vi "VariantToByteArray.vi"(8 "error in":errorcluster, 9 "bytearray_in":u8[](array[numeric]), 11 "variant":variant) -> (0 "error out":errorcluster, 3 "byte_array_out[]":u8[](array[numeric]))   [LabVIEW 2020]
uses:
  <vilib>/Utility/Data Type/NI_Data Type.lvlib
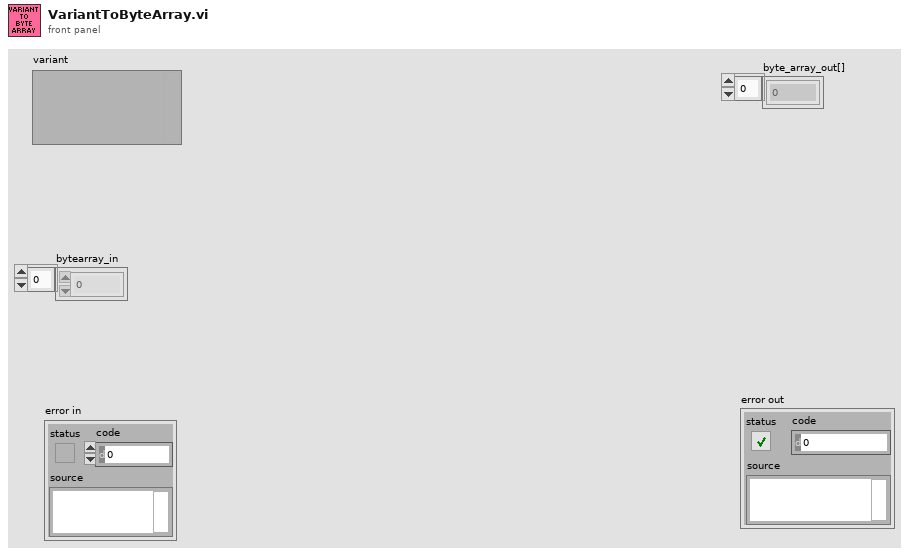
[diagram p1: front panel]
types:
  T1 = typedef "NI_Data Type.lvlib/Data Type.ctl" = enum8{"Invalid Type", "Void", "I8", "I16", "I32", "I64", "U8", "U16", "U32", "U64", "Single Float", "Double Float", "Extended Float", "Single Complex", "Double Complex", "Extended Complex", "Enum U8", "Enum U16", "Enum U32", "Enum U64", "Single Float With Unit", "Double Float With Unit", "Extended Float With Unit", "Single Complex with Unit", "Double Complex with Unit", "Extended Complex with Unit", "Boolean", "String", "Path", "Picture", "Tag", "Array", "Cluster", "Variant", "LV Variant", "Waveform", "Timestamp", "Digital Waveform", "Digital Data", "ExpressData", "Refnum", "External Data", "VI", "Poly VI", "LabVIEW Class Instance", "Fixed Point", "Set Collection", "Map Collection"}
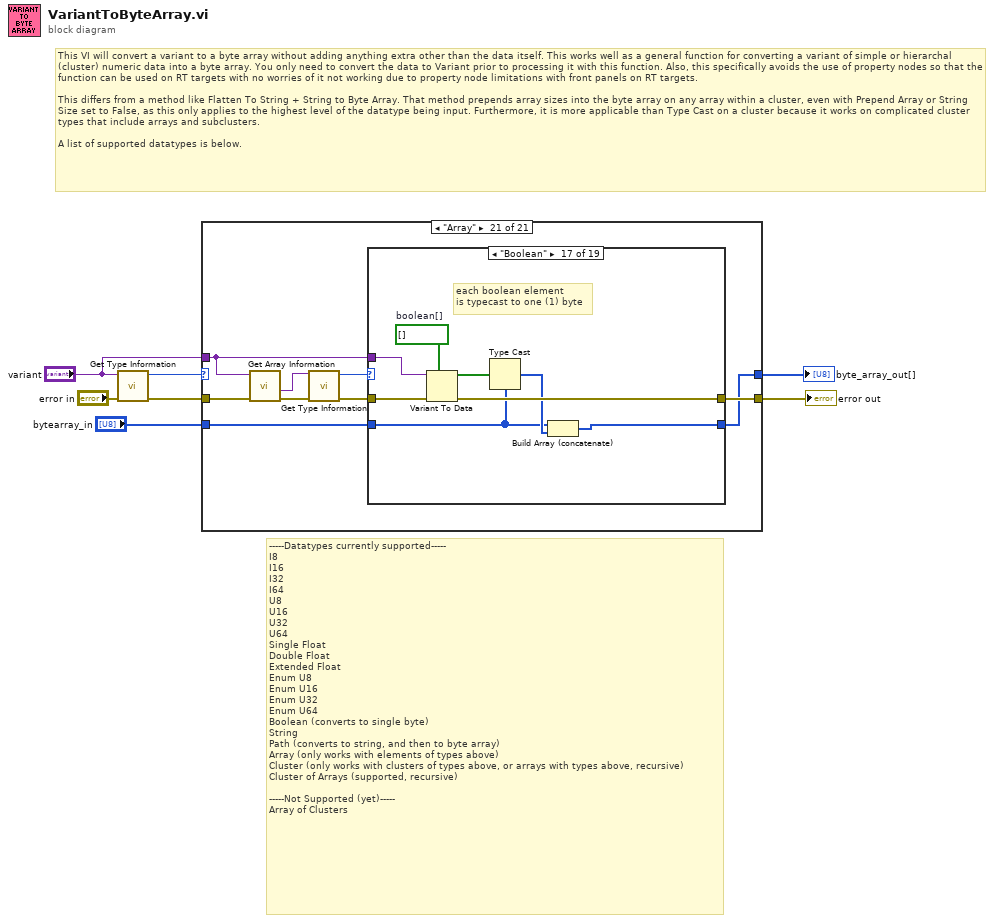
[diagram p0: block diagram]
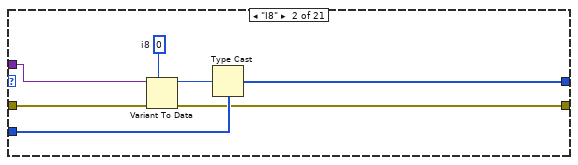
[diagram p3: hidden frame]
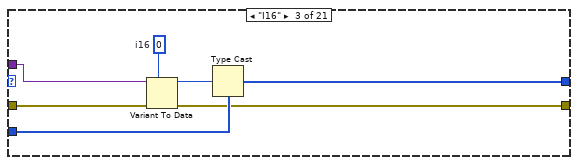
[diagram p4: hidden frame]
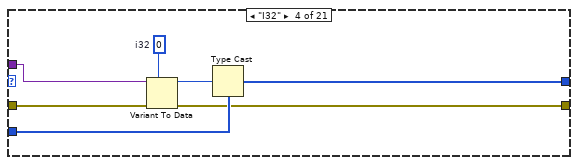
[diagram p5: hidden frame]
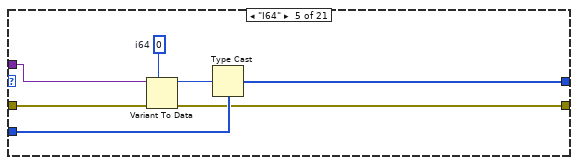
[diagram p6: hidden frame]
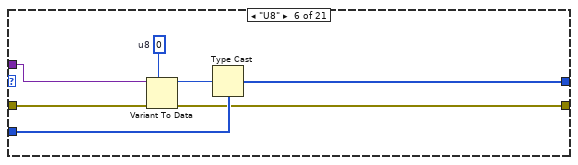
[diagram p7: hidden frame]
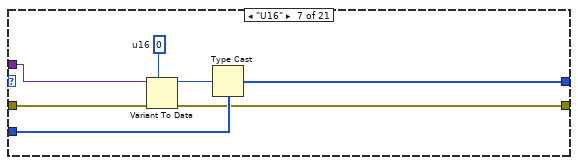
[diagram p8: hidden frame]
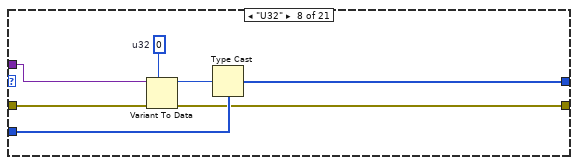
[diagram p9: hidden frame]
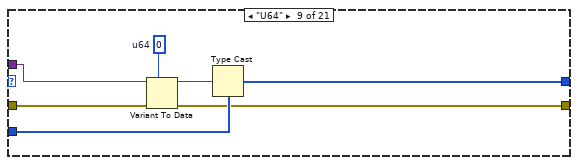
[diagram p10: hidden frame]
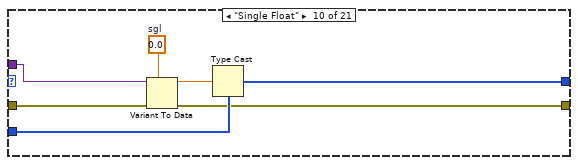
[diagram p11: hidden frame]
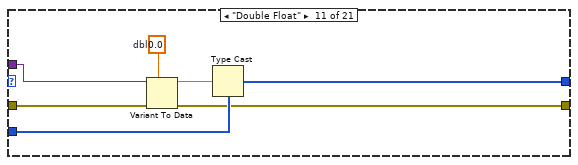
[diagram p12: hidden frame]
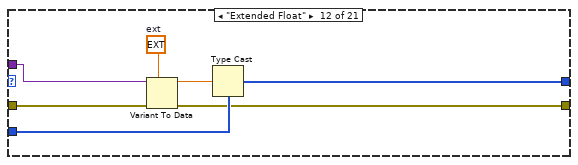
[diagram p13: hidden frame]
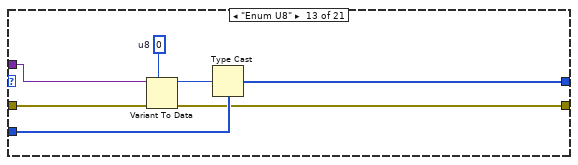
[diagram p14: hidden frame]
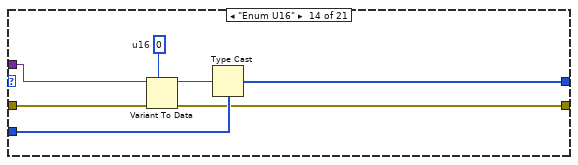
[diagram p15: hidden frame]
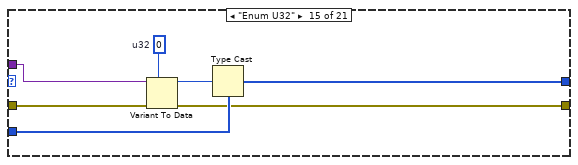
[diagram p16: hidden frame]
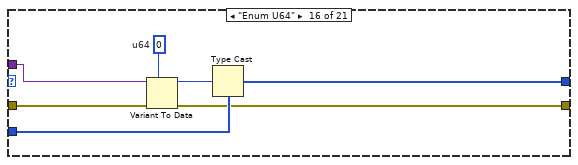
[diagram p17: hidden frame]
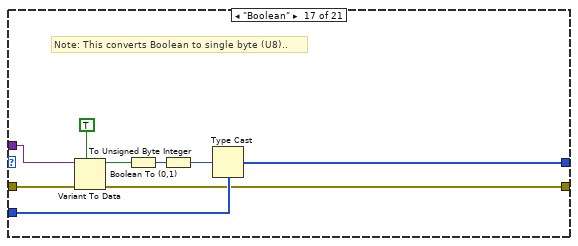
[diagram p18: hidden frame]
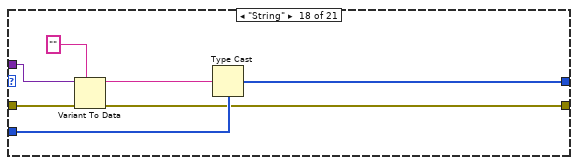
[diagram p19: hidden frame]
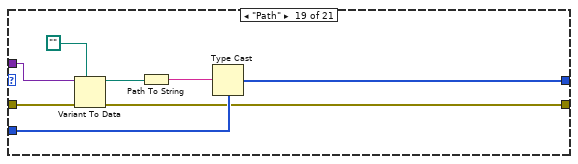
[diagram p20: hidden frame]
diagram:
  # "This VI will convert a variant to a byte array without adding anything extra other than the data itself. This works well as a general function for converting a variant of simple or hierarchal (cluster) numeric data into a byte array. You only need to convert the data to Variant prior to processing it with this function. Also, this specifically avoids the use of property nodes so that the function can be used on RT targets with no worries of it not working due to property node limitations with front panels on RT targets.\n\nThis differs from a method like Flatten To String + String to Byte Array. That method prepends array sizes into the byte array on any array within a cluster, even with Prepend Array or String Size set to False, as this only applies to the highest level of the datatype being input. Furthermore, it is more applicable than Type Cast on a cluster because it works on complicated cluster types that include arrays and subclusters.\n\nA list of supported datatypes is below."
  # "-----Datatypes currently supported-----\nI8\nI16\nI32\nI64\nU8\nU16\nU32\nU64\nSingle Float\nDouble Float\nExtended Float\nEnum U8\nEnum U16\nEnum U32\nEnum U64\nBoolean (converts to single byte)\nString\nPath (converts to string, and then to byte array)\nArray (only works with elements of types above)\nCluster (only works with clusters of types above, or arrays with types above, recursive) \nCluster of Arrays (supported, recursive)\n\n-----Not Supported (yet)-----\nArray of Clusters"
  n1 = call <vilib>:"Get Type Information.vi"("error in (no error)"="error in", "variant"="variant") -> ("error out"=w6:errorcluster, "type"=w7:T1)  [unwired: 5 in, 3 out]
  n2 = case shown="\"Array\"" w7 {
    tunnel: "variant" -> [_ w16 w23 w30 w37 w44 w51 w58 w65 w72 w79 w86 w93 w100 w107 w114 w123 w130 w138 w145 w155]
    tunnel: [w8 w13 w20 w27 w34 w41 w48 w55 w62 w69 w76 w83 w90 w97 w104 w111 w121 w129 w137 w140 w154] -> w1
    tunnel: "bytearray_in" -> [w8 w12 w19 w26 w33 w40 w47 w54 w61 w68 w75 w82 w89 w96 w103 w110 w120 w128 w136 w141 w157]
    tunnel: w6 -> [w9 w11 w18 w25 w32 w39 w46 w53 w60 w67 w74 w81 w88 w95 w102 w109 w119 w127 w135 w144 w161]
    tunnel: [w9 w10 w17 w24 w31 w38 w45 w52 w59 w66 w73 w80 w87 w94 w101 w108 w118 w126 w134 w139 w162] -> w2
    frame "Invalid Type", Default {
    }
    frame "I8" {
      w14 = i8 0  # i8
      n3 = Variant To Data(error in=w11, type=w14, Variant=w16) -> (data=w15:i8, error out=w10:errorcluster)
      n4 = Type Cast(type=w12, x=w15) -> (*(type *) &x=w13:u8[])
    }
    frame "I16" {
      w21 = i16 0  # i16
      n5 = Variant To Data(error in=w18, type=w21, Variant=w23) -> (data=w22:i16, error out=w17:errorcluster)
      n6 = Type Cast(type=w19, x=w22) -> (*(type *) &x=w20:u8[])
    }
    frame "I32" {
      w28 = 0  # i32
      n7 = Variant To Data(error in=w25, type=w28, Variant=w30) -> (data=w29:i32, error out=w24:errorcluster)
      n8 = Type Cast(type=w26, x=w29) -> (*(type *) &x=w27:u8[])
    }
    frame "I64" {
      w35 = i64 0  # i64
      n9 = Variant To Data(error in=w32, type=w35, Variant=w37) -> (data=w36:i64, error out=w31:errorcluster)
      n10 = Type Cast(type=w33, x=w36) -> (*(type *) &x=w34:u8[])
    }
    frame "U8" {
      w42 = u8 0  # u8
      n11 = Variant To Data(error in=w39, type=w42, Variant=w44) -> (data=w43:u8, error out=w38:errorcluster)
      n12 = Type Cast(type=w40, x=w43) -> (*(type *) &x=w41:u8[])
    }
    frame "U16" {
      w49 = u16 0  # u16
      n13 = Variant To Data(error in=w46, type=w49, Variant=w51) -> (data=w50:u16, error out=w45:errorcluster)
      n14 = Type Cast(type=w47, x=w50) -> (*(type *) &x=w48:u8[])
    }
    frame "U32" {
      w56 = u32 0  # u32
      n15 = Variant To Data(error in=w53, type=w56, Variant=w58) -> (data=w57:u32, error out=w52:errorcluster)
      n16 = Type Cast(type=w54, x=w57) -> (*(type *) &x=w55:u8[])
    }
    frame "U64" {
      w63 = u64 0  # u64
      n17 = Variant To Data(error in=w60, type=w63, Variant=w65) -> (data=w64:u64, error out=w59:errorcluster)
      n18 = Type Cast(type=w61, x=w64) -> (*(type *) &x=w62:u8[])
    }
    frame "Single Float" {
      w70 = sgl 0.0  # sgl
      n19 = Variant To Data(error in=w67, type=w70, Variant=w72) -> (data=w71:sgl, error out=w66:errorcluster)
      n20 = Type Cast(type=w68, x=w71) -> (*(type *) &x=w69:u8[])
    }
    frame "Double Float" {
      w77 = 0.0  # dbl
      n21 = Variant To Data(error in=w74, type=w77, Variant=w79) -> (data=w78:dbl, error out=w73:errorcluster)
      n22 = Type Cast(type=w75, x=w78) -> (*(type *) &x=w76:u8[])
    }
    frame "Extended Float" {
      w84 = ext 0.0  # ext
      n23 = Variant To Data(error in=w81, type=w84, Variant=w86) -> (data=w85:ext, error out=w80:errorcluster)
      n24 = Type Cast(type=w82, x=w85) -> (*(type *) &x=w83:u8[])
    }
    frame "Enum U8" {
      w91 = u8 0  # u8
      n25 = Variant To Data(error in=w88, type=w91, Variant=w93) -> (data=w92:u8, error out=w87:errorcluster)
      n26 = Type Cast(type=w89, x=w92) -> (*(type *) &x=w90:u8[])
    }
    frame "Enum U16" {
      w98 = u16 0  # u16
      n27 = Variant To Data(error in=w95, type=w98, Variant=w100) -> (data=w99:u16, error out=w94:errorcluster)
      n28 = Type Cast(type=w96, x=w99) -> (*(type *) &x=w97:u8[])
    }
    frame "Enum U32" {
      w105 = u32 0  # u32
      n29 = Variant To Data(error in=w102, type=w105, Variant=w107) -> (data=w106:u32, error out=w101:errorcluster)
      n30 = Type Cast(type=w103, x=w106) -> (*(type *) &x=w104:u8[])
    }
    frame "Enum U64" {
      w112 = u64 0  # u64
      n31 = Variant To Data(error in=w109, type=w112, Variant=w114) -> (data=w113:u64, error out=w108:errorcluster)
      n32 = Type Cast(type=w110, x=w113) -> (*(type *) &x=w111:u8[])
    }
    frame "Boolean" {
      # "Note: This converts Boolean to single byte (U8).."
      n33 = Variant To Data(error in=w119, type=TRUE, Variant=w123) -> (data=w117:bool, error out=w118:errorcluster)
      n34 = Boolean To (0,1)(Boolean=w117) -> (0, 1=w115:i16)
      n35 = To Unsigned Byte Integer(number=w115) -> (unsigned 8bit integer=w116:u8)
      n36 = Type Cast(type=w120, x=w116) -> (*(type *) &x=w121:u8[])
    }
    frame "String" {
      n37 = Variant To Data(error in=w127, type="", Variant=w130) -> (data=w124:string, error out=w126:errorcluster)
      n38 = Type Cast(type=w128, x=w124) -> (*(type *) &x=w129:u8[])
    }
    frame "Path" {
      n39 = Variant To Data(error in=w135, type=path "", Variant=w138) -> (data=w132:path, error out=w134:errorcluster)
      n40 = Path To String(path=w132) -> (string=w131:string)
      n41 = Type Cast(type=w136, x=w131) -> (*(type *) &x=w137:u8[])
    }
    frame "Cluster" {
      n42 = call <vilib>:"Get Cluster Information.vi"("error in (no error)"=w144, "variant"=w145) -> ("error out"=w146:errorcluster, "cluster elements"=w147:variant[])  [unwired: 8 in]
      n43 = Variant To Data(error in=w146, type=w147, Variant=w145) -> (data=w142:variant[], error out=w143:errorcluster)
      n44 = for {
        shift-right: [w151] -> w139
        shift-left: w143 -> [w153]
        tunnel: w142 -> [w152] mode=indexing
        shift-right: [w148] -> w140
        shift-left: w141 -> [w149]
        n45 = call "VariantToByteArray.vi"("error in"=w153, "variant"=w152) -> ("error out"=w151:errorcluster, "byte_array_out[]"=w150:u8[])  [unwired: 8 in]
        n46 = Build Array (concatenate)(w149, w150) -> (w148:u8[])
      }
    }
    frame "Array" {
      n47 = call <vilib>:"Get Array Information.vi"("error in (no error)"=w161, "variant"=w155) -> ("error out"=w160:errorcluster, "array element data type"=w159:variant)  [unwired: 6 in, 2 out]
      n48 = call <vilib>:"Get Type Information.vi"("error in (no error)"=w160, "variant"=w159) -> ("error out"=w156:errorcluster, "type"=w158:T1)  [unwired: 5 in, 3 out]
      n49 = case shown="\"Boolean\"" w158 {
        tunnel: w157 -> [w164 w165 w173 w181 w189 w198 w204 w212 w220 w228 w236 w244 w252 w260 w268 w276 w284 w293 w306]
        tunnel: w156 -> [w163 w171 w179 w187 w195 w202 w210 w218 w226 w234 w242 w250 w258 w266 w274 w282 w290 w301 w314]
        tunnel: w155 -> [_ w170 w178 w186 w194 w201 w209 w217 w225 w233 w241 w249 w257 w265 w273 w281 w289 w300 w313]
        tunnel: [w164 w167 w175 w183 w191 w199 w206 w214 w222 w230 w238 w246 w254 w262 w270 w278 w286 w298 w311] -> w154
        tunnel: [w163 w172 w180 w188 w196 w203 w211 w219 w227 w235 w243 w251 w259 w267 w275 w283 w291 w292 w305] -> w162
        frame "Invalid Type", Default {
        }
        frame "I8" {
          w169 = i8[] []  # i8[]
          n50 = Variant To Data(error in=w171, type=w169, Variant=w170) -> (data=w168:i8[], error out=w172:errorcluster)
          n51 = Type Cast(type=w165, x=w168) -> (*(type *) &x=w166:u8[])
          n52 = Build Array (concatenate)(w165, w166) -> (w167:u8[])
        }
        frame "I16" {
          w177 = i16[] []  # i16[]
          n53 = Variant To Data(error in=w179, type=w177, Variant=w178) -> (data=w176:i16[], error out=w180:errorcluster)
          n54 = Type Cast(type=w173, x=w176) -> (*(type *) &x=w174:u8[])
          n55 = Build Array (concatenate)(w173, w174) -> (w175:u8[])
        }
        frame "I32" {
          w185 = i32[] []  # i32[]
          n56 = Variant To Data(error in=w187, type=w185, Variant=w186) -> (data=w184:i32[], error out=w188:errorcluster)
          n57 = Type Cast(type=w181, x=w184) -> (*(type *) &x=w182:u8[])
          n58 = Build Array (concatenate)(w181, w182) -> (w183:u8[])
        }
        frame "I64" {
          w193 = i64[] []  # i64[]
          n59 = Variant To Data(error in=w195, type=w193, Variant=w194) -> (data=w192:i64[], error out=w196:errorcluster)
          n60 = Type Cast(type=w189, x=w192) -> (*(type *) &x=w190:u8[])
          n61 = Build Array (concatenate)(w189, w190) -> (w191:u8[])
        }
        frame "U8" {
          w200 = u8[] []  # u8[]
          n62 = Variant To Data(error in=w202, type=w200, Variant=w201) -> (data=w197:u8[], error out=w203:errorcluster)
          n63 = Build Array (concatenate)(w198, w197) -> (w199:u8[])
        }
        frame "U16" {
          w208 = u16[] []  # u16[]
          n64 = Variant To Data(error in=w210, type=w208, Variant=w209) -> (data=w207:u16[], error out=w211:errorcluster)
          n65 = Type Cast(type=w204, x=w207) -> (*(type *) &x=w205:u8[])
          n66 = Build Array (concatenate)(w204, w205) -> (w206:u8[])
        }
        frame "U32" {
          w216 = u32[] []  # u32[]
          n67 = Variant To Data(error in=w218, type=w216, Variant=w217) -> (data=w215:u32[], error out=w219:errorcluster)
          n68 = Type Cast(type=w212, x=w215) -> (*(type *) &x=w213:u8[])
          n69 = Build Array (concatenate)(w212, w213) -> (w214:u8[])
        }
        frame "U64" {
          w224 = u64[] []  # u64[]
          n70 = Variant To Data(error in=w226, type=w224, Variant=w225) -> (data=w223:u64[], error out=w227:errorcluster)
          n71 = Type Cast(type=w220, x=w223) -> (*(type *) &x=w221:u8[])
          n72 = Build Array (concatenate)(w220, w221) -> (w222:u8[])
        }
        frame "Single Float" {
          w232 = sgl[] []  # sgl[]
          n73 = Variant To Data(error in=w234, type=w232, Variant=w233) -> (data=w231:sgl[], error out=w235:errorcluster)
          n74 = Type Cast(type=w228, x=w231) -> (*(type *) &x=w229:u8[])
          n75 = Build Array (concatenate)(w228, w229) -> (w230:u8[])
        }
        frame "Double Float" {
          w240 = dbl[] []  # dbl[]
          n76 = Variant To Data(error in=w242, type=w240, Variant=w241) -> (data=w239:dbl[], error out=w243:errorcluster)
          n77 = Type Cast(type=w236, x=w239) -> (*(type *) &x=w237:u8[])
          n78 = Build Array (concatenate)(w236, w237) -> (w238:u8[])
        }
        frame "Extended Float" {
          w248 = ext[] []  # ext[]
          n79 = Variant To Data(error in=w250, type=w248, Variant=w249) -> (data=w247:ext[], error out=w251:errorcluster)
          n80 = Type Cast(type=w244, x=w247) -> (*(type *) &x=w245:u8[])
          n81 = Build Array (concatenate)(w244, w245) -> (w246:u8[])
        }
        frame "Enum U8" {
          w256 = u8[] []  # u8[]
          n82 = Variant To Data(error in=w258, type=w256, Variant=w257) -> (data=w255:u8[], error out=w259:errorcluster)
          n83 = Type Cast(type=w252, x=w255) -> (*(type *) &x=w253:u8[])
          n84 = Build Array (concatenate)(w252, w253) -> (w254:u8[])
        }
        frame "Enum U16" {
          w264 = u16[] []  # u16[]
          n85 = Variant To Data(error in=w266, type=w264, Variant=w265) -> (data=w263:u16[], error out=w267:errorcluster)
          n86 = Type Cast(type=w260, x=w263) -> (*(type *) &x=w261:u8[])
          n87 = Build Array (concatenate)(w260, w261) -> (w262:u8[])
        }
        frame "Enum U32" {
          w272 = u32[] []  # u32[]
          n88 = Variant To Data(error in=w274, type=w272, Variant=w273) -> (data=w271:u32[], error out=w275:errorcluster)
          n89 = Type Cast(type=w268, x=w271) -> (*(type *) &x=w269:u8[])
          n90 = Build Array (concatenate)(w268, w269) -> (w270:u8[])
        }
        frame "Enum U64" {
          w280 = u64[] []  # u64[]
          n91 = Variant To Data(error in=w282, type=w280, Variant=w281) -> (data=w279:u64[], error out=w283:errorcluster)
          n92 = Type Cast(type=w276, x=w279) -> (*(type *) &x=w277:u8[])
          n93 = Build Array (concatenate)(w276, w277) -> (w278:u8[])
        }
        frame "Boolean" {
          w288 = bool[] []  # boolean[]
          # "each boolean element\nis typecast to one (1) byte"
          n94 = Variant To Data(error in=w290, type=w288, Variant=w289) -> (data=w287:bool[], error out=w291:errorcluster)
          n95 = Type Cast(type=w284, x=w287) -> (*(type *) &x=w285:u8[])
          n96 = Build Array (concatenate)(w284, w285) -> (w286:u8[])
        }
        frame "String" {
          w299 = string[] []  # string[]
          n97 = Variant To Data(error in=w301, type=w299, Variant=w300) -> (data=w296:string[], error out=w292:errorcluster)
          n98 = for {
            tunnel: w296 -> [w304] mode=indexing
            shift-right: [w302] -> w294
            shift-left: "" -> [w303]
            n99 = Concatenate Strings(w303, w304) -> (w302:string)
          }
          n100 = String To Byte Array(string=w294) -> (unsigned byte array=w297:u8[])
          n101 = Build Array (concatenate)(w293, w297) -> (w298:u8[])
        }
        frame "Path" {
          w312 = path[] []  # path[]
          n102 = Variant To Data(error in=w314, type=w312, Variant=w313) -> (data=w309:path[], error out=w305:errorcluster)
          n103 = for {
            tunnel: w309 -> [w316] mode=indexing
            shift-right: [w317] -> w307
            shift-left: "" -> [w318]
            n104 = Path To String(path=w316) -> (string=w315:string)
            n105 = Concatenate Strings(w318, w315) -> (w317:string)
          }
          n106 = String To Byte Array(string=w307) -> (unsigned byte array=w310:u8[])
          n107 = Build Array (concatenate)(w306, w310) -> (w311:u8[])
        }
      }
    }
  }
  "byte_array_out[]" <- w1
  "error out" <- w2
